vi "Program List with Home_R3.vi"(7 "Model":string, 8 "error in":errorcluster, 9 "FeedBack Channel":string[](array[string])=["fgdgfvcbc", "vnfhgjkn", "21354682"], 10 "Filepath":path=path "D:/My Project/2019-2020/Magnetic Mareli UM/MM_UM/Project Setup/data/program seq/Program_280A.bin", 11 "vi referenceIn":refnum<vi>) -> (0 "error out":errorcluster, 1 "Exit":bool, 2 "String":string, 3 "vi reference Out":refnum<vi>)   [LabVIEW 2015]
uses:
  Control Button/Exit.ctl
  Control Button/next.ctl
  Galobal variable_TI.vi
panel:
  out "String 2":string
  in  "Next":T1
  in  "Exit":T2
  in  "Program List":string(combo)
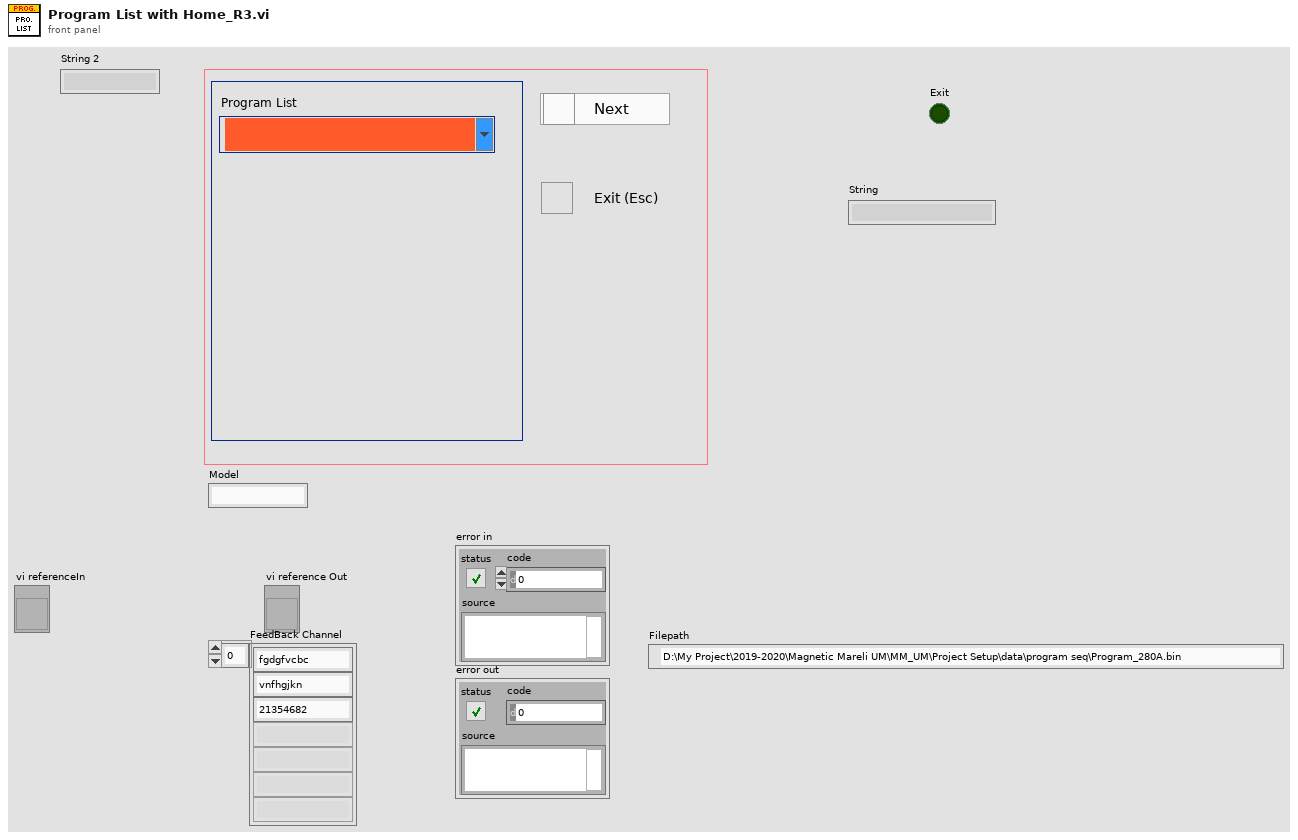
[diagram p1: front panel]
types:
  T1 = typedef "next.ctl" = bool
  T2 = typedef "Exit.ctl" = bool
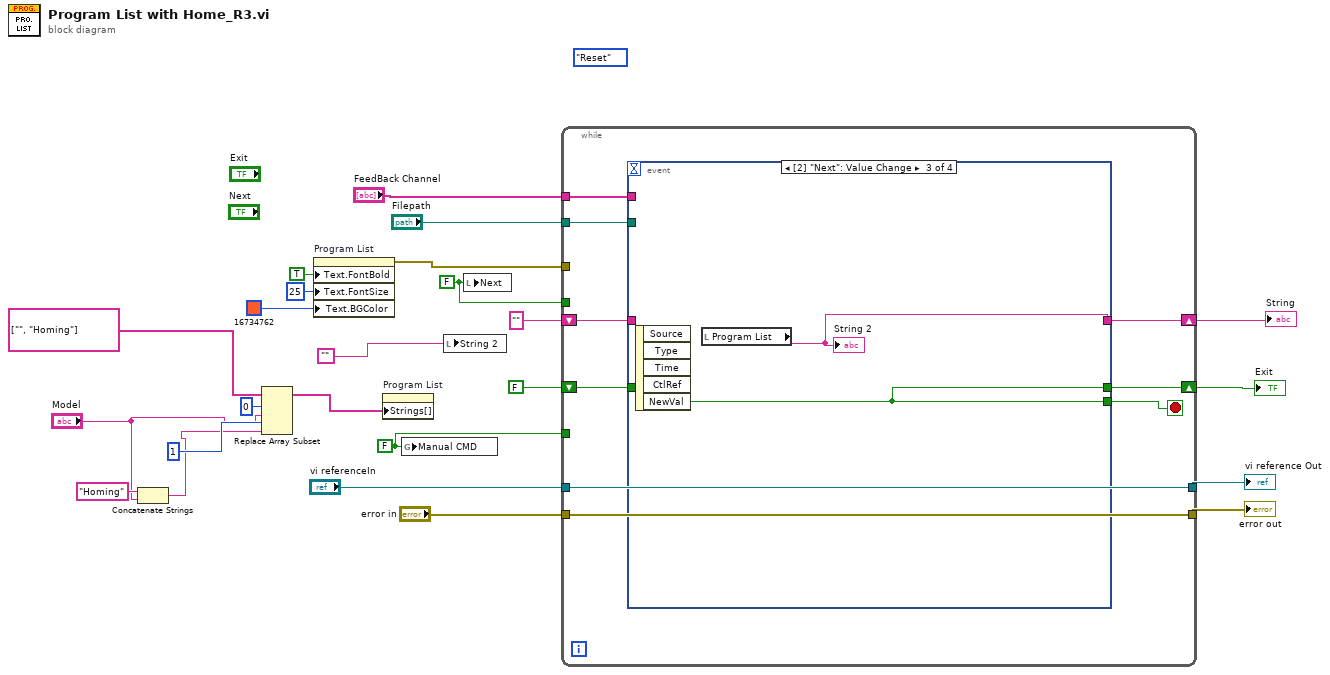
[diagram p0: block diagram]
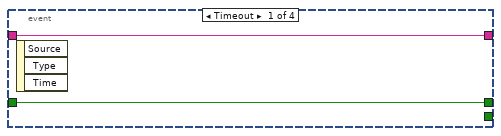
[diagram p2: hidden frame]
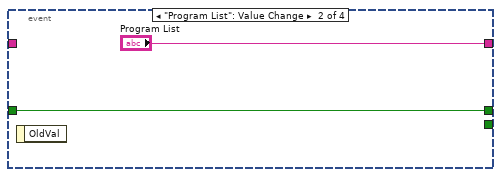
[diagram p3: hidden frame]
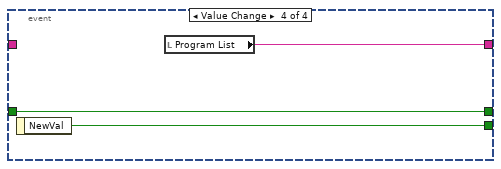
[diagram p4: hidden frame]
diagram:
  (unwired) enum16{"Home", "Reset"}."Reset"
  w14 = FALSE ("Manual CMD")
  w15 = FALSE ("Next")
  n1 = Concatenate Strings("Homing" ("string"), "Model") -> (w2:string)
  n2 = Replace Array Subset(array=string[] ["", "Homing"] ("Strings []"), new element #1="Model", index #1=0 ("index"), new element #2=w2, index #2=1 ("index")) -> (w6:string[])
  n3 = property on="Program List" class="CmbBox"("Text.FontBold"=TRUE ("Text.Font:Bold"), "Text.FontSize"=u32 25 ("Text.Font:Size"), "Text.BGColor"=u32 16734762 ("Color Box")) -> (error out=w18:errorcluster)  [unwired: 2 in, 1 out]
  n4 = property on="Program List" class="CmbBox"("Strings[]"=w6) -> ()  [unwired: 2 in, 2 out]
  n5 = global write "Galobal variable_TI.vi" "Manual CMD"(w14) -> ()
  n6 = local write "String 2"("") -> ()
  n7 = local write "Next"(w15) -> ()
  n8 = while {
    shift-right: [w33] -> w24
    shift-left: "" ("Combo Box") -> [w32]
    shift-right: [w30] -> w21
    shift-left: T2 FALSE ("NewVal") -> [w29]
    tunnel: w18 -> [_]
    tunnel: w15 -> [_]
    tunnel: w14 -> [_]
    tunnel: "vi referenceIn" -> [w28]
    tunnel: [w28] -> w12
    tunnel: "error in" -> [w27]
    tunnel: [w27] -> w10
    tunnel: "Filepath" -> [w26]
    tunnel: "FeedBack Channel" -> [w25]
    stop <- w31 stop-if-true
    n9 = event shown="[2] \"Next\": Value Change" {
      selector: _ -> [_ _ _ _]
      dyn-events: _ -> [_ _ _ _]
      timeout: _ -> [_ _ _ _]
      tunnel: [w35 "Program List" w38 w41] -> w33
      tunnel: w32 -> [w35 _ _ _]
      tunnel: [_ _ w39 w42] -> w31
      tunnel: [w34 w36 w39 w40] -> w30
      tunnel: w29 -> [w34 w36 _ w40]
      tunnel: w26 -> [_ _ _ _]
      tunnel: w25 -> [_ _ _ _]
      event Timeout {
        n10 = event-data() -> ()  [unwired: 1 in, 3 out]
      }
      event "Program List": Value Change {
        n11 = event-data() -> ()  [unwired: 1 in, 1 out]
      }
      event Value Change {
        n12 = event-data() -> ("NewVal"=w39:T1)  [unwired: 1 in, 4 out]
        n13 = local read "Program List"() -> (w38:string)
        "String 2" <- w38
      }
      event Value Change {
        n14 = event-data() -> ("NewVal"=w42:T2)  [unwired: 1 in]
        n15 = local read "Program List"() -> (w41:string)
      }
    }
  }
  "String" <- w24
  "Exit" <- w21
  "vi reference Out" <- w12
  "error out" <- w10
